vi "back_prop.vi"(5 "Expected Output":dbl, 6 "Learning Parameter":dbl, 7 "Output":dbl, 9 "Biases":cluster{dbl[], dbl[], dbl[]}, 10 "Weights":cluster{dbl[][], dbl[][], dbl[][]}, 11 "Data Output":cluster{"Input":dbl[], "1H":dbl[], dbl[]}) -> (3 "output cluster":T1)   [LabVIEW 2018]
panel:
  # "2H"
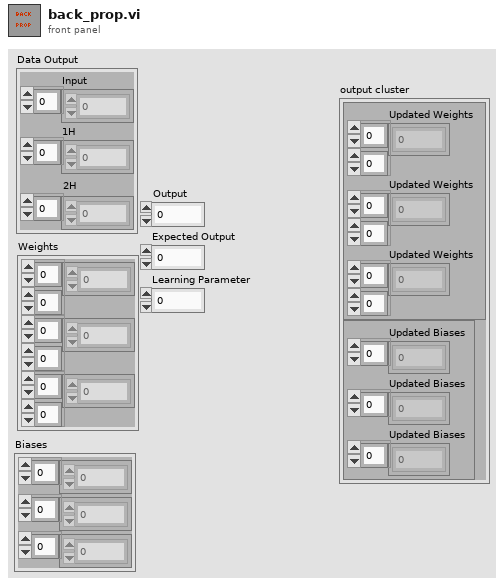
[diagram p1: front panel]
types:
  T1 = cluster{cluster{"Updated Weights":dbl[][], "Updated Weights":dbl[][], "Updated Weights":dbl[][]}, cluster{"Updated Biases":dbl[], "Updated Biases":dbl[], "Updated Biases":dbl[]}}
  T2 = cluster{"Updated Biases":dbl[], "Updated Biases":dbl[], "Updated Biases":dbl[]}
  T3 = cluster{"Updated Weights":dbl[][], "Updated Weights":dbl[][], "Updated Weights":dbl[][]}
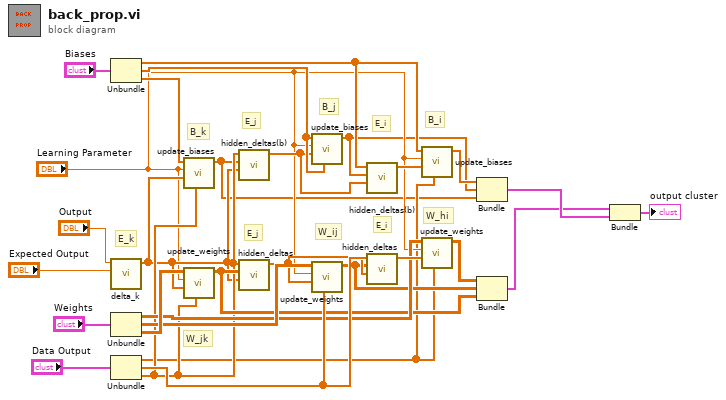
[diagram p0: block diagram]
diagram:
  # "B_i"
  # "E_i"
  # "B_j"
  # "E_j"
  # "B_k"
  # "W_hi"
  # "E_i"
  # "W_ij"
  # "E_k"
  # "E_j"
  # "W_jk"
  n1 = Unbundle("Biases") -> (w7:dbl[], w10:dbl[], w13:dbl[])
  n2 = call "delta_k.vi"("Expected Output"="Expected Output", "Output"="Output") -> ("Delta K"=w11:dbl[])  [unwired: 9 in]
  n3 = Unbundle("Weights") -> (w17:dbl[][], w21:dbl[][], w22:dbl[][])
  n4 = Unbundle("Data Output") -> ("Input"=w5:dbl[], "1H"=w20:dbl[], w12:dbl[])
  n5 = call "update_biases.vi"("Back Output"=w12, "Delta"=w11, "Learning Parameter"="Learning Parameter", "Biases"=w13) -> ("Updated Biases"=w2:dbl[])  [unwired: 7 in]
  n6 = call "update_weights.vi"("Back Output"=w12, "Delta"=w11, "Learning Parameter"="Learning Parameter", "Weights"=w22) -> ("Updated Weights"=w14:dbl[][])  [unwired: 7 in]
  n7 = call "hidden_deltas(b).vi"("Forward Delta"=w11, "Forward Biases"=w2, "Node Outputs"=w12) -> ("Current Delta"=w9:dbl[])  [unwired: 8 in]
  n8 = call "hidden_deltas.vi"("Forward Delta"=w11, "Forward Weights"=w14, "Node Outputs"=w12) -> ("Current delta"=w19:dbl[])  [unwired: 8 in]
  n9 = call "update_biases.vi"("Back Output"=w10, "Delta"=w9, "Learning Parameter"="Learning Parameter", "Biases"=w10) -> ("Updated Biases"=w3:dbl[])  [unwired: 7 in]
  n10 = call "update_weights.vi"("Back Output"=w20, "Delta"=w19, "Learning Parameter"="Learning Parameter", "Weights"=w21) -> ("Updated Weights"=w15:dbl[][])  [unwired: 7 in]
  n11 = call "hidden_deltas(b).vi"("Forward Delta"=w9, "Forward Biases"=w3, "Node Outputs"=w7) -> ("Current Delta"=w8:dbl[])  [unwired: 8 in]
  n12 = call "hidden_deltas.vi"("Forward Delta"=w19, "Forward Weights"=w15, "Node Outputs"=w20) -> ("Current delta"=w18:dbl[])  [unwired: 8 in]
  n13 = call "update_biases.vi"("Back Output"=w5, "Delta"=w8, "Learning Parameter"="Learning Parameter", "Biases"=w7) -> ("Updated Biases"=w4:dbl[])  [unwired: 7 in]
  n14 = call "update_weights.vi"("Back Output"=w5, "Delta"=w18, "Learning Parameter"="Learning Parameter", "Weights"=w17) -> ("Updated Weights"=w16:dbl[][])  [unwired: 7 in]
  n15 = Bundle("Updated Biases"=w4, "Updated Biases"=w3, "Updated Biases"=w2) -> (w27:T2)  [unwired: 1 in]
  n16 = Bundle("Updated Weights"=w16, "Updated Weights"=w15, "Updated Weights"=w14) -> (w26:T3)  [unwired: 1 in]
  n17 = Bundle(w26, w27) -> (→"output cluster":T1)  [unwired: 1 in]
